vi "Oscop 2 Channel Phase Diff.vi"(7 "Perform Auto Setup":bool, 8 "error in (no error)":errorcluster, 11 "VISA resource name":refnum<visa-resource-name>) -> (0 "error out":errorcluster, 2 "Value":dbl format="%#_3f", 3 "VISA resource name out":refnum<visa-resource-name>)   [LabVIEW 2021]
uses:
  Program Files/National Instruments/LabVIEW 2021/instr.lib/Siglent SDS 1000 2000 Series/Siglent SDS 1000 2000 Series.lvlib
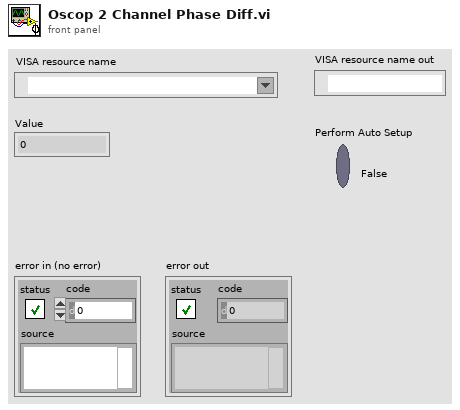
[diagram p1: front panel]
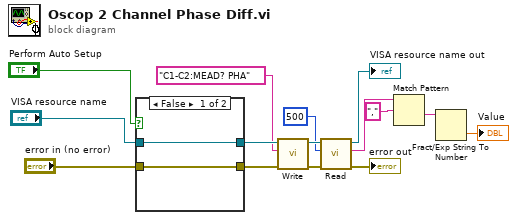
[diagram p0: block diagram]
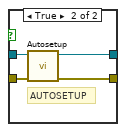
[diagram p2: hidden frame]
diagram:
  n1 = case shown="False" "Perform Auto Setup" {
    tunnel: "error in (no error)" -> [w16 w21]
    tunnel: "VISA resource name" -> [w17 w20]
    tunnel: [w17 w19] -> w8
    tunnel: [w16 w18] -> w7
    frame False {
    }
    frame True {
      # "AUTOSETUP"
      n2 = call "Autosetup.vi"("error in (no error)"=w21, "VISA resource name"=w20) -> ("error out"=w18:errorcluster, "VISA resource name out"=w19:refnum<visa-resource-name>)  [unwired: 8 in]
    }
  }
  n3 = call "Write.vi"("error in (no error)"=w7, "Write Buffer"="C1-C2:MEAD? PHA", "VISA resource name"=w8) -> ("error out"=w9:errorcluster, "VISA resource name out"=w12:refnum<visa-resource-name>)  [unwired: 6 in, 1 out]
  n4 = call "Read.vi"("error in (no error)"=w9, "Byte Count"=u32 500, "VISA resource name"=w12) -> ("error out"=→"error out":errorcluster, "Read Buffer"=w1:string, "VISA resource name out"=→"VISA resource name out":refnum<visa-resource-name>)  [unwired: 5 in, 1 out]
  n5 = Match Pattern(string=w1, regular expression=",") -> (after substring=w3:string)  [unwired: 1 in, 3 out]
  n6 = Fract/Exp String To Number(string=w3) -> (number=→"Value":dbl)  [unwired: 3 in, 1 out]
